vi "RetrievePix.vi"(11 "RawDataFile":path) -> (0 "CamSelect":bool[](array[boolean]), 1 "PicPath":T1(array[cluster]), 2 "CamNames":string[](array[string]))   [LabVIEW 2022 SP3]
panel:
  in  "fullSize":bool
  out "loaded?":bool
  in  "Reload":bool
  in  "CamSelectIn":bool[](array[boolean])=[TRUE, TRUE, TRUE, TRUE]
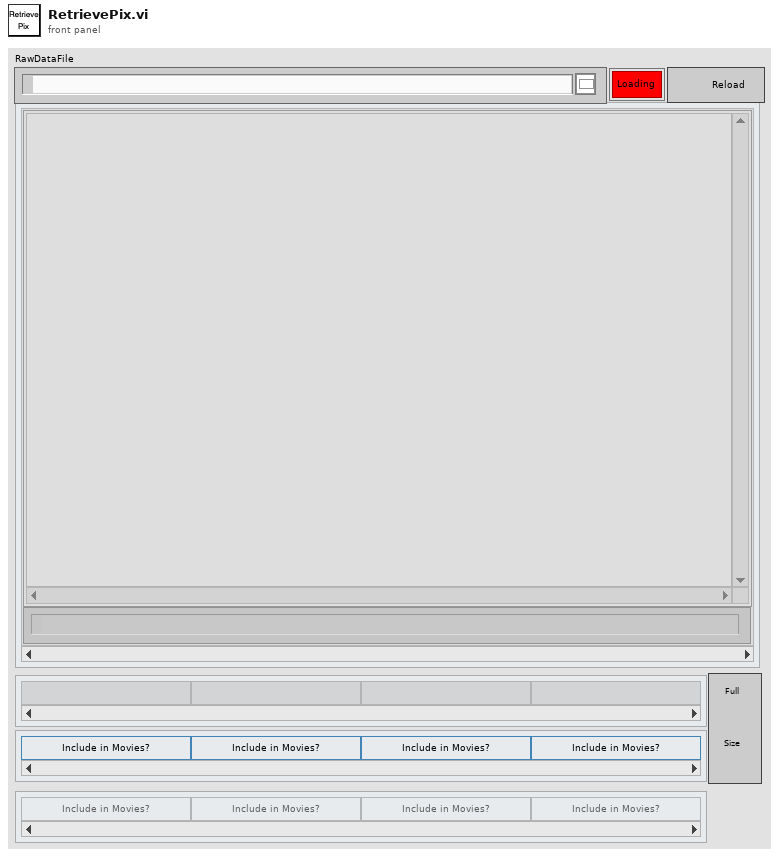
[diagram p1: front panel]
types:
  T1 = cluster{"new picture":picture, "image path":path}[]
  T2 = typedef "imagedata.ctl" = cluster{"image type":i32, "image depth":i32, "image":u8[], "mask":u8[], "colors":u32[], "Rectangle":cluster{"left":i16, "top":i16, "right":i16, "bottom":i16}}
  T3 = cluster{"new picture":picture, "appended path":path}
  T4 = cluster{"new picture":picture, "appended path":path}[]
  T5 = cluster{"missingPicture":picture, "appended path":path}
  T6 = cluster{"missingPicture":picture, "appended path":path}[]
  T7 = typedef "LVRectTypeDef.ctl" = cluster{"Left":i16, "Top":i16, "Right":i16, "Bottom":i16}
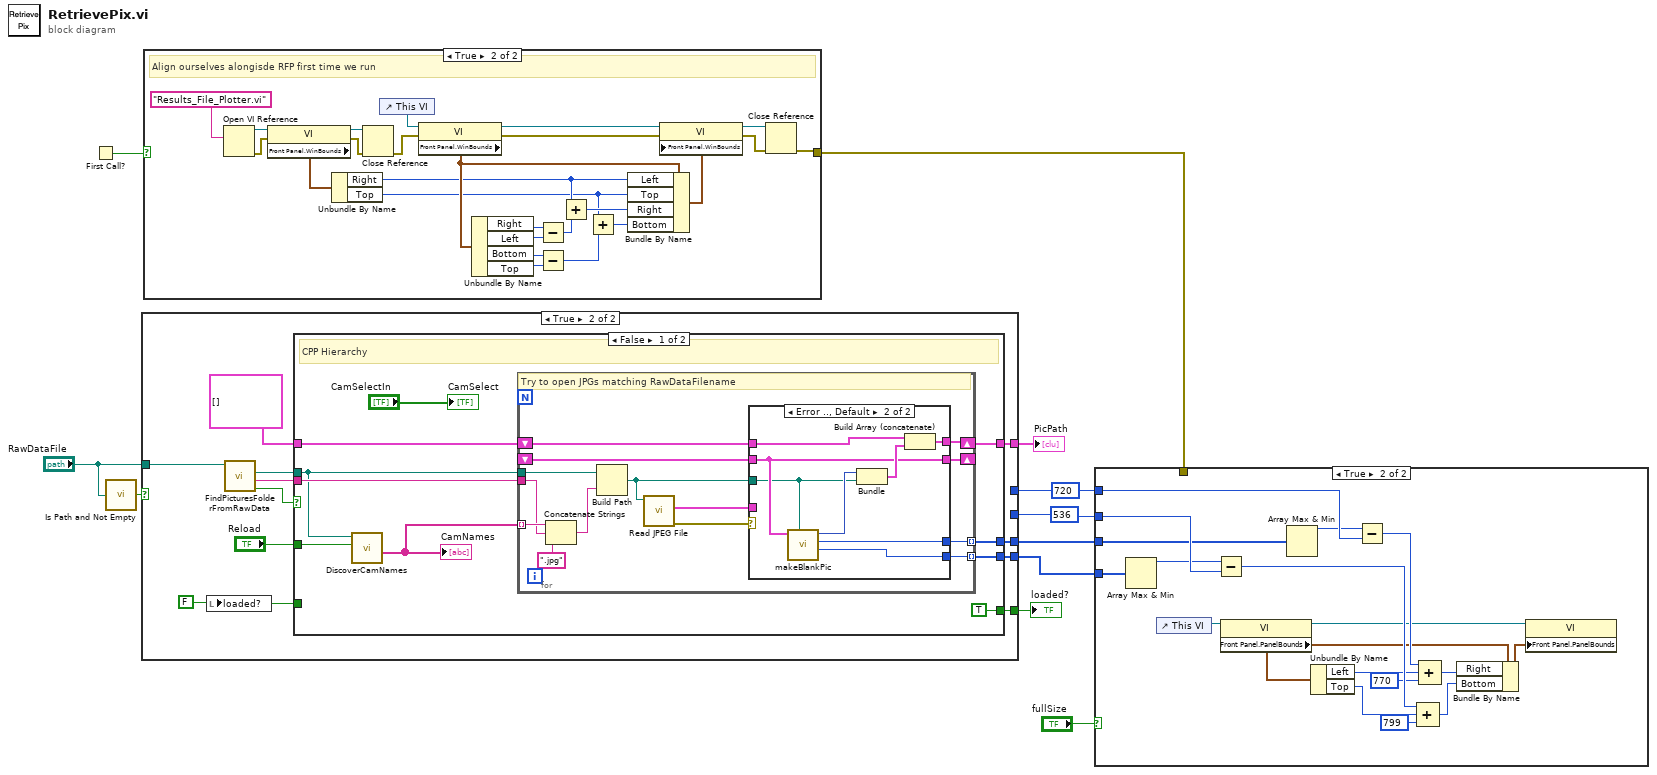
[diagram p0: block diagram]
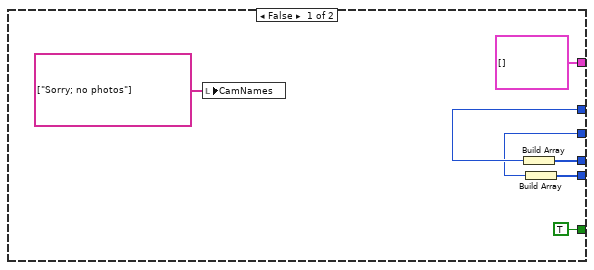
[diagram p3: hidden frame]
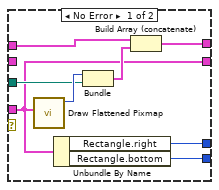
[diagram p4: hidden frame]
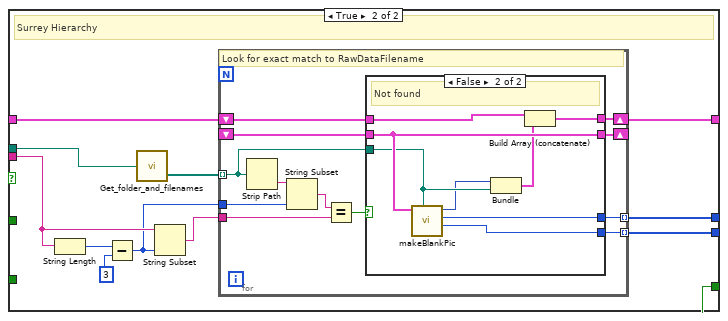
[diagram p5: hidden frame]
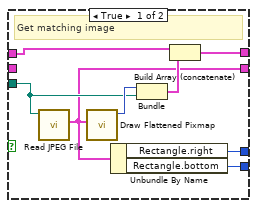
[diagram p6: hidden frame]
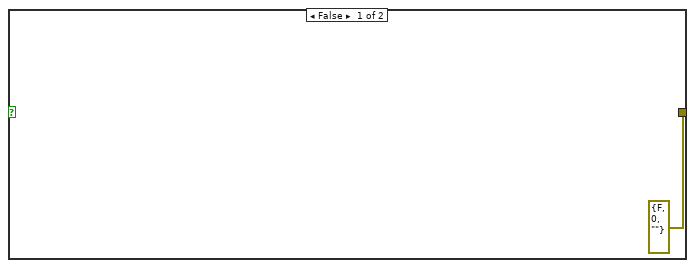
[diagram p7: hidden frame]
diagram:
  w1 = 536
  w2 = 720
  n1 = First Call?() -> (First Call?: T/F=w7:bool)
  n2 = call <vilib>:"Is Path and Not Empty.vi"("path"="RawDataFile") -> ("Is Path and Not Empty?"=w10:bool)  [unwired: 4 in]
  n3 = case shown="True" w10 {
    tunnel: "RawDataFile" -> [_ w29]
    tunnel: [T1 [] ("Array 2") w24] -> w8
    tunnel: [TRUE ("loaded?") w22] -> w11
    tunnel: [w15 w20] -> w5
    tunnel: [w14 w19] -> w6
    tunnel: w2 -> [w13 _]
    tunnel: w1 -> [w12 _]
    frame False {
      n4 = local write "CamNames"(string[] ["Sorry; no photos"] ("CamNames")) -> ()
      n5 = Build Array(w13) -> (w15:i32[])
      n6 = Build Array(w12) -> (w14:i32[])
    }
    frame True {
      w21 = FALSE
      n7 = local write "loaded?"(w21) -> ()
      n8 = call "FindPicturesFolderFromRawData.vi"("RawDataFile"=w29) -> ("SurreyPath?"=w26:bool, "RawDataName"=w27:string, "PicturesPath"=w28:path)  [unwired: 8 in]
      n9 = case shown="False" w26 {
        tunnel: [w38 w74] -> w24
        tunnel: w28 -> [w37 w81]
        tunnel: w27 -> [w39 w77]
        tunnel: "Reload" -> [w36 _]
        tunnel: T1 [] ("Array 2") -> [w35 w73]
        tunnel: [TRUE ("loaded?") TRUE ("loaded?")] -> w22
        tunnel: w21 -> [_ _]
        tunnel: [w31 w71] -> w20
        tunnel: [w30 w70] -> w19
        frame False {
          # "CPP Hierarchy"
          n10 = call "DiscoverCamNames.vi"("Rescan"=w36, "PicturesPath"=w37) -> ("CamNames"=w34:string[])  [unwired: 9 in]
          "CamNames" <- w34
          n11 = for {
            tunnel: w39 -> [w48]
            shift-right: [w52] -> w38
            shift-left: w35 -> [w53]
            tunnel: w37 -> [w51]
            tunnel: w34 -> [w49] mode=indexing
            tunnel: [w44] -> w31 mode=indexing
            tunnel: [w43] -> w30 mode=indexing
            shift-right: [w41] -> _
            shift-left: _ -> [w40]
            # "Try to open JPGs matching RawDataFilename"
            n12 = Concatenate Strings(w49, w48, ".jpg" ("string")) -> (w46:string)
            n13 = Build Path(base path=w51, name or relative path=w46) -> (appended path=w50:path)
            n14 = call <vilib>:"Read JPEG File.vi"("path to JPEG file"=w50) -> ("error out"=w45:errorcluster, "image data"=w42:T2)  [unwired: 8 in, 1 out]
            n15 = case shown="Error .., Default" w45 {
              tunnel: w53 -> [w61 w69]
              tunnel: [w60 w68] -> w52
              tunnel: w42 -> [w54 _]
              tunnel: w50 -> [w57 w62]
              tunnel: [w56 w65] -> w44
              tunnel: [w55 w64] -> w43
              tunnel: w40 -> [_ w63]
              tunnel: [w54 w63] -> w41
              frame No Error {
                n16 = call <vilib>:"Draw Flattened Pixmap.vi"("image data"=w54) -> ("new picture"=w59:picture)  [unwired: 8 in]
                n17 = Unbundle By Name(w54) -> ("Rectangle.right"=w56:i16, "Rectangle.bottom"=w55:i16)
                n18 = Bundle("new picture"=w59, "appended path"=w57) -> (w58:T3)  [unwired: 1 in]
                n19 = Build Array (concatenate)(w61, w58) -> (w60:T4)
              }
              frame Error, Default {
                n20 = call "makeBlankPic.vi"("File Path"=w62, "previousImageData"=w63) -> ("bottom"=w64:i16, "right"=w65:i16, "missingPicture"=w67:picture)  [unwired: 7 in]
                n21 = Bundle("missingPicture"=w67, "appended path"=w62) -> (w66:T5)  [unwired: 1 in]
                n22 = Build Array (concatenate)(w69, w66) -> (w68:T6)
              }
            }
          }
          "CamSelect" <- "CamSelectIn"
        }
        frame True {
          # "Surrey Hierarchy"
          n23 = String Length(string=w77) -> (length=w79:i32)
          n24 = Subtract(x=w79, y=3) -> (x-y=w76:i32)
          n25 = call "Get_folder_and_filenames.vi"("file path (dialog if empty)"=w81) -> ("Files"=w80:path[])  [unwired: 1 out]
          n26 = String Subset(string=w77, length (rest)=w76) -> (substring=w75:string)  [unwired: 1 in]
          n27 = for {
            shift-right: [w92] -> w74
            shift-left: w73 -> [w93]
            tunnel: w80 -> [w86] mode=indexing
            tunnel: w76 -> [w90]
            tunnel: w75 -> [w87]
            tunnel: [w85] -> w71 mode=indexing
            tunnel: [w84] -> w70 mode=indexing
            shift-right: [w83] -> _
            shift-left: _ -> [w82]
            # "Look for exact match to RawDataFilename"
            n28 = Strip Path(path=w86) -> (name=w91:string)  [unwired: 1 out]
            n29 = String Subset(string=w91, length (rest)=w90) -> (substring=w89:string)  [unwired: 1 in]
            n30 = Equal?(x=w89, y=w87) -> (x = y?=w88:bool)
            n31 = case shown="False" w88 {
              tunnel: w93 -> [w101 w104]
              tunnel: [w100 w105] -> w92
              tunnel: w86 -> [w97 w103]
              tunnel: [w96 w108] -> w85
              tunnel: [w95 w107] -> w84
              tunnel: [w94 w109] -> w83
              tunnel: w82 -> [_ w109]
              frame True {
                # "Get matching image"
                n32 = call <vilib>:"Read JPEG File.vi"("path to JPEG file"=w97) -> ("image data"=w94:T2)  [unwired: 8 in, 2 out]
                n33 = call <vilib>:"Draw Flattened Pixmap.vi"("image data"=w94) -> ("new picture"=w98:picture)  [unwired: 8 in]
                n34 = Unbundle By Name(w94) -> ("Rectangle.right"=w96:i16, "Rectangle.bottom"=w95:i16)
                n35 = Bundle("new picture"=w98, "appended path"=w97) -> (w99:T3)  [unwired: 1 in]
                n36 = Build Array (concatenate)(w101, w99) -> (w100:T4)
              }
              frame False {
                # "Not found"
                n37 = call "makeBlankPic.vi"("File Path"=w103, "previousImageData"=w109) -> ("bottom"=w107:i16, "right"=w108:i16, "missingPicture"=w102:picture)  [unwired: 7 in]
                n38 = Bundle("missingPicture"=w102, "appended path"=w103) -> (w106:T5)  [unwired: 1 in]
                n39 = Build Array (concatenate)(w104, w106) -> (w105:T6)
              }
            }
          }
        }
      }
    }
  }
  "PicPath" <- w8
  "loaded?" <- w11
  n40 = case shown="True" w7 {
    tunnel: [errorcluster {"status"=FALSE, "code"=0, "source"=""} ("error out") w111] -> w3
    frame False {
    }
    frame True {
      # "Align ourselves alongisde RFP first time we run"
      n41 = Open VI Reference(vi path="Results_File_Plotter.vi") -> (vi reference=w134:refnum<vi>, error out=w123:errorcluster)  [unwired: 5 in]
      n42 = property class="VI"(reference=w134, error in=w123) -> (reference out=w128:refnum<vi>, error out=w127:errorcluster, "Front Panel.WinBounds"=w132:T7)
      n43 = Unbundle By Name(w132) -> ("Right"=w116:i16, "Top"=w113:i16)
      n44 = Close Reference(reference=w128, error in (no error)=w127) -> (error out=w126:errorcluster)
      n45 = control-ref of="This VI"() -> (w133:refnum<vi>)
      n46 = property class="VI"(reference=w133, error in=w126) -> (reference out=w130:refnum<vi>, error out=w125:errorcluster, "Front Panel.WinBounds"=w122:T7)
      n47 = Unbundle By Name(w122) -> ("Right"=w121:i16, "Left"=w120:i16, "Bottom"=w119:i16, "Top"=w118:i16)
      n48 = Subtract(x=w121, y=w120) -> (x-y=w117:i16)
      n49 = Subtract(x=w119, y=w118) -> (x-y=w114:i16)
      n50 = Add(x=w116, y=w117) -> (x+y=w115:i16)
      n51 = Add(x=w113, y=w114) -> (x+y=w112:i16)
      n52 = Bundle By Name(cluster=w122, "Left"=w116, "Top"=w113, "Right"=w115, "Bottom"=w112) -> (w131:T7)
      n53 = property class="VI"(reference=w130, error in=w125, "Front Panel.WinBounds"=w131) -> (reference out=w129:refnum<vi>, error out=w124:errorcluster)
      n54 = Close Reference(reference=w129, error in (no error)=w124) -> (error out=w111:errorcluster)
    }
  }
  n55 = case shown="True" "fullSize" {
    tunnel: w2 -> [_ w151]
    tunnel: w1 -> [_ w150]
    tunnel: w6 -> [_ w149]
    tunnel: w5 -> [_ w136]
    tunnel: w3 -> [_ _]
    frame False {
    }
    frame True {
      n56 = Array Max & Min(array=w149) -> (max value=w138:i32)  [unwired: 3 out]
      n57 = control-ref of="This VI"() -> (w148:refnum<vi>)
      n58 = Subtract(x=w138, y=w150) -> (x-y=w152:i32)
      n59 = property class="VI"(reference=w148) -> (reference out=w147:refnum<vi>, "Front Panel.PanelBounds"=w143:T7)  [unwired: 1 in, 1 out]
      n60 = Array Max & Min(array=w136) -> (max value=w137:i32)  [unwired: 3 out]
      n61 = Unbundle By Name(w143) -> ("Left"=w142:i16, "Top"=w140:i16)
      n62 = Subtract(x=w137, y=w151) -> (x-y=w153:i32)
      n63 = Compound Arithmetic op=ADD(w152, w140, i16 799 ("value")) -> (w144:i32)
      n64 = Compound Arithmetic op=ADD(w153, w142, i16 770 ("value")) -> (w145:i32)
      n65 = Bundle By Name(cluster=w143, "Right"=w145, "Bottom"=w144) -> (w146:T7)
      n66 = property class="VI"(reference=w147, "Front Panel.PanelBounds"=w146) -> ()  [unwired: 1 in, 2 out]
    }
  }
